vi "Generate Valid Test Numbers.vi"(0 "Session Handle in":T4, 5 "Include All Evaluations?":bool=TRUE, 7 "Test Group":string, 9 "Evaluations In":T1[](array[typedef]) {"Low Limit" format="%#_13g"; "SI Scaling" items=["femto"=-15, "pico"=-12, "nano"=-9, "micro"=-6, "milli"=-3, "percent"=-2, ""=0, "kilo"=3, "mega"=6, "giga"=9, "tera"=12]}, 11 "error in (no error)":errorcluster) -> (4 "Session Handle out":T4, 10 "Evaluations Out":T1[](array[typedef]) {"Low Limit" format="%#_13g"; "SI Scaling" items=["femto"=-15, "pico"=-12, "nano"=-9, "micro"=-6, "milli"=-3, "percent"=-2, ""=0, "kilo"=3, "mega"=6, "giga"=9, "tera"=12]}, 15 "error out":errorcluster)   [LabVIEW 2018, in "Test Number and Bin Generator.lvlib" / "Test Number and Bin Generator.lvclass"]
uses:
  Test Number and Bin Generator.lvclass
  Typedefs/Session Handle.ctl
  Plugins/TestStand API Tools (TSAT).lvlibp/Evaluation Actions/Includes/Controls/TSAT Evaluation.ctl
  Plugins/TestStand API Tools (TSAT).lvlibp/Evaluation Actions/Includes/Controls/TSAT Eval SI Unit Scaling.ctl
  Plugins/TestStand API Tools (TSAT).lvlibp/Evaluation Actions/Includes/Controls/TSAT Evaluation Type.ctl
  Test Number and Bin Generator.lvclass/Test Number and Bin Generator.ctl
  Test Group/Test Group.lvclass
  Test Group/Test Group.lvclass/Test Group.ctl
  Plugins/TestStand API Tools (TSAT).lvlibp/Evaluation Actions/TSAT Evaluation Actions.lvlib
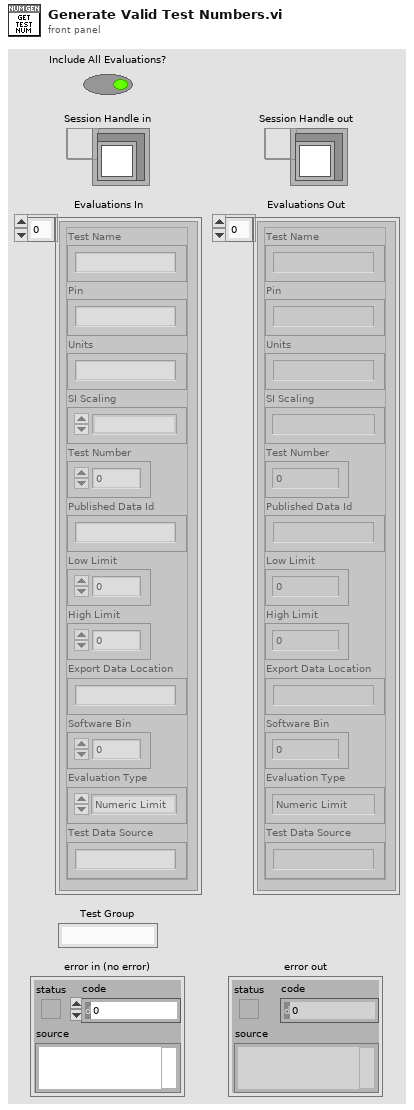
[diagram p1: front panel]
types:
  T1 = typedef "TestStand API Tools (TSAT).lvlibp/TSAT Evaluation Actions.lvlib/TSAT Evaluation.ctl" = cluster{"Test Name":string, "Pin":string, "Units":string, "SI Scaling":T2, "Test Number":i32, "Published Data Id":string, "Low Limit":dbl, "High Limit":dbl, "Export Data Location":string, "Software Bin":i64, "Evaluation Type":T3, "Test Data Source":string}
  T2 = typedef "TestStand API Tools (TSAT).lvlibp/TSAT Evaluation Actions.lvlib/TSAT Eval SI Unit Scaling.ctl" = i16
  T3 = typedef "TestStand API Tools (TSAT).lvlibp/TSAT Evaluation Actions.lvlib/TSAT Evaluation Type.ctl" = enum16{"Numeric Limit", "Pass/Fail", "None"}
  T4 = typedef "Test Number and Bin Generator.lvlib/Test Number and Bin Generator.lvclass/Session Handle.ctl" = refnum<data-value>
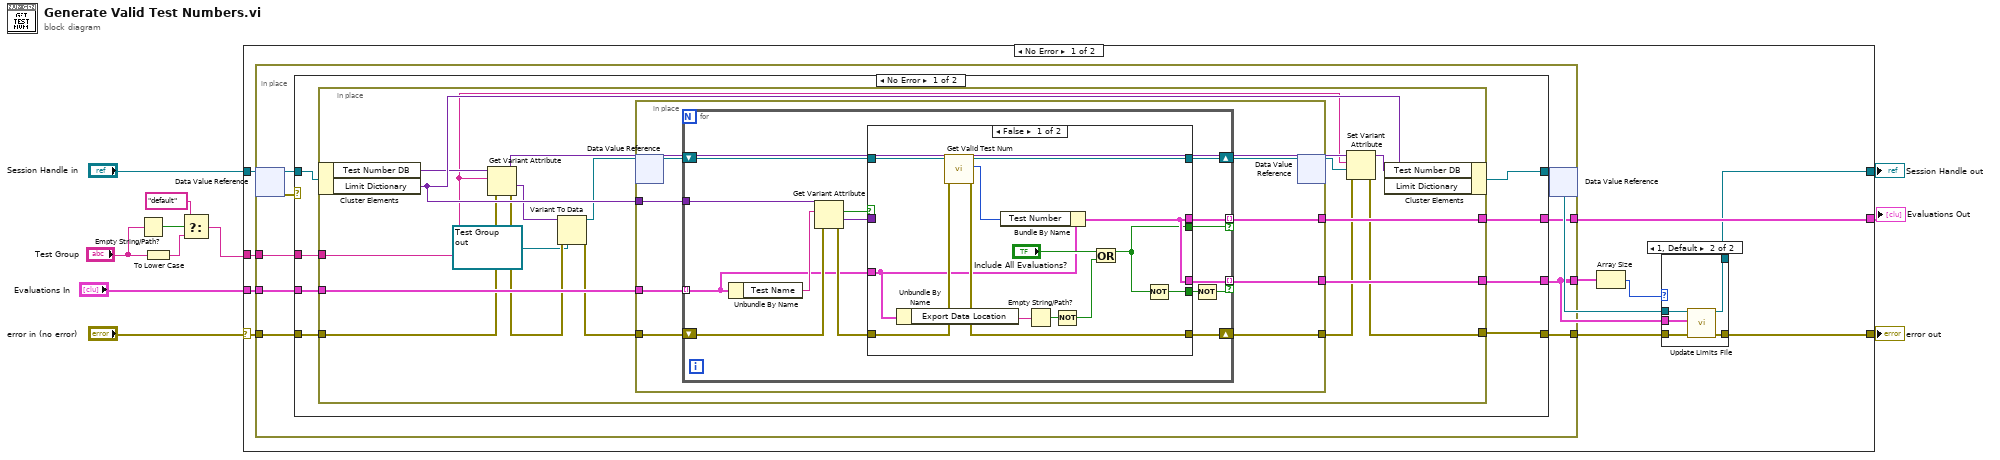
[diagram p0: block diagram]
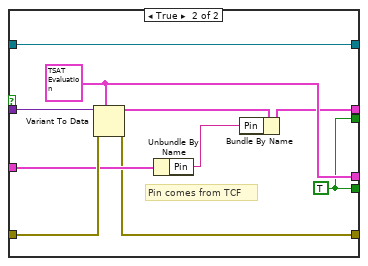
[diagram p3: hidden frame]
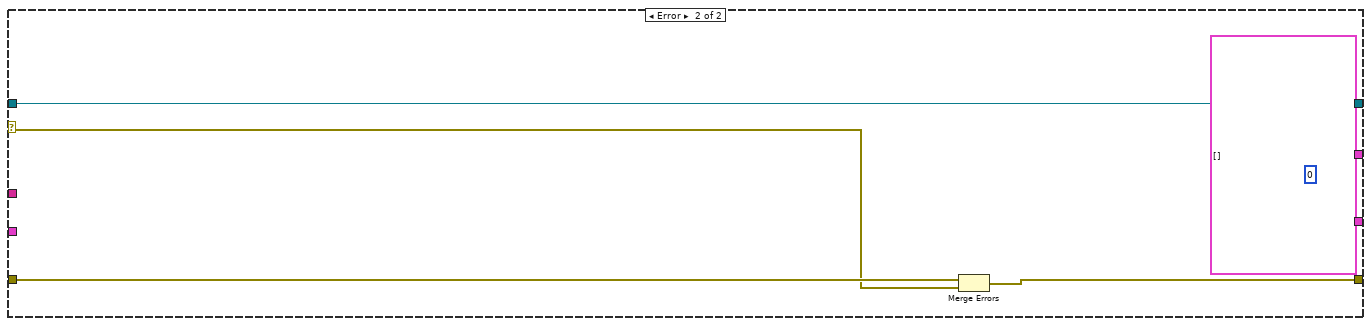
[diagram p4: hidden frame]
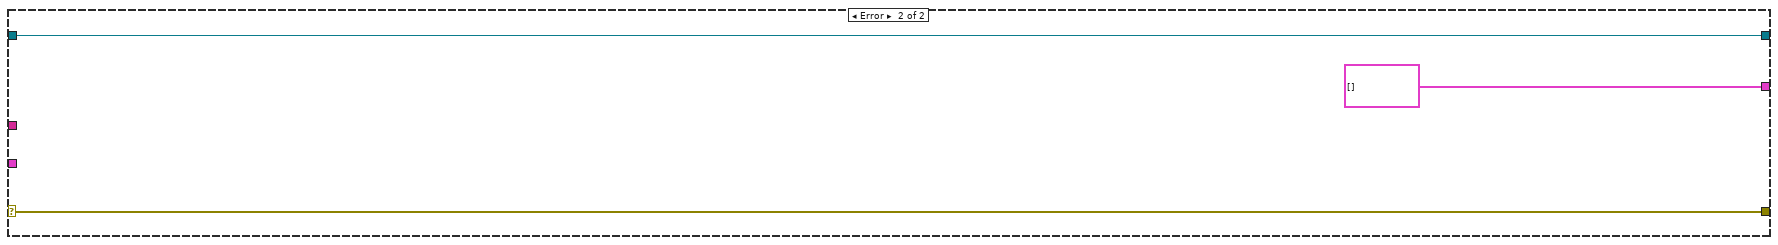
[diagram p5: hidden frame]
diagram:
  n1 = Empty String/Path?(string/path="Test Group") -> (empty?=w5:bool)
  n2 = To Lower Case(string="Test Group") -> (all lower case string=w2:string)
  n3 = Select(t="default", s=w5, f=w2) -> (s? t:f=w1:string)
  n4 = case shown="No Error" "error in (no error)" {
    selector: "error in (no error)" -> [w21 w116]
    tunnel: "Session Handle in" -> [w22 w117]
    tunnel: [w12 w117] -> w10
    tunnel: [w15 w116] -> w9
    tunnel: w1 -> [w20 _]
    tunnel: "Evaluations In" -> [w19 _]
    tunnel: [w18 T1[] []] -> w6
    frame No Error {
      n5 = in-place {
        in-place-border: w21 -> [w34]
        in-place-border: [w37] -> w16
        in-place-border: w20 -> [w33]
        in-place-border: w19 -> [w32]
        in-place-border: [w31] -> w18
        in-place-border: [w30] -> w14
        n6 = in-place-dvr #1(w22) -> (w38:refnum<class "Test Number and Bin Generator.lvclass">, w35:errorcluster)
        n7 = case shown="No Error" w35 {
          selector: w35 -> [_ w113]
          tunnel: w38 -> [w46 w111]
          tunnel: [w42 w112] -> w37
          tunnel: [w45 w111] -> w36
          tunnel: w34 -> [w44 w114]
          tunnel: w33 -> [w43 _]
          tunnel: w32 -> [w41 _]
          tunnel: [w40 w110] -> w31
          tunnel: [w39 w110] -> w30
          frame No Error {
            n8 = in-place {
              in-place-border: w44 -> [w59]
              in-place-border: w43 -> [w49]
              in-place-border: [w53] -> w42
              in-place-border: w41 -> [w63]
              in-place-border: [w62] -> w40
              in-place-border: [w61] -> w39
              n9 = in-place-cluster #2(w46) -> ("Test Number DB"=w58:variant, "Limit Dictionary"=w60:variant)
              n10 = Get Variant Attribute(Variant=w58, name=w49, error in=w59) -> (duplicate Variant=w50:variant, value=w47:variant, error out=w57:errorcluster)  [unwired: 1 in, 1 out]
              n11 = Variant To Data(error in=w57, type=refnum<data-value> refnum ("data value reference"), Variant=w47) -> (data=w55:refnum<data-value>, error out=w56:errorcluster)
              n12 = in-place {
                in-place-border: w63 -> [w71]
                in-place-border: [w70] -> w52
                in-place-border: [w69] -> w62
                in-place-border: [w68] -> w61
                in-place-border: w60 -> [w67]
                in-place-border: w56 -> [w66]
                n13 = in-place-dvr #3(w55) -> (w65:refnum<class "Test Group.lvclass">)  [unwired: 1 out]
                n14 = for {
                  tunnel: w71 -> [w79] mode=indexing
                  shift-right: [w78] -> w70
                  shift-left: w66 -> [w84]
                  tunnel: [w80] -> w69 mode=indexing if=w72
                  tunnel: [w77] -> w68 mode=indexing if=w75
                  tunnel: w67 -> [w86]
                  shift-right: [w73] -> w64
                  shift-left: w65 -> [w74]
                  n15 = Unbundle By Name(w79) -> ("Test Name"=w85:string)
                  n16 = Get Variant Attribute(Variant=w86, name=w85, error in=w84) -> (found=w83:bool, value=w81:variant, error out=w82:errorcluster)  [unwired: 1 in, 1 out]
                  n17 = case shown="False" w83 {
                    tunnel: w82 -> [w95 w107]
                    tunnel: w81 -> [_ w109]
                    tunnel: [w99 w102] -> w80
                    tunnel: w79 -> [w91 w104]
                    tunnel: [w94 w100] -> w78
                    tunnel: [w99 w108] -> w77
                    tunnel: [w92 w105] -> w76
                    tunnel: w74 -> [w98 w106]
                    tunnel: [w96 w106] -> w73
                    tunnel: [w89 w105] -> w72
                    frame False {
                      n18 = Unbundle By Name(w91) -> ("Export Data Location"=w90:string)
                      n19 = call "Get Valid Test Num.vi"("error in (no error)"=w95, "Test Group in"=w98) -> ("error out"=w94:errorcluster, "Numeric"=w97:i32, "Test Group out"=w96:refnum<class "Test Group.lvclass">)  [unwired: 7 in]
                      n20 = Bundle By Name(cluster=w91, "Test Number"=w97) -> (w99:T1)
                      n21 = Empty String/Path?(string/path=w90) -> (empty?=w88:bool)
                      n22 = Not(x=w88) -> (.not. x?=w87:bool)
                      n23 = Or(x="Include All Evaluations?", y=w87) -> (x .or. y?=w89:bool)
                      n24 = Not(x=w89) -> (.not. x?=w92:bool)
                    }
                    frame True {
                      w105 = TRUE
                      w108 = T1 {"Test Name"="", "Pin"="", "Units"="", "SI Scaling"=0, "Test Number"=0, "Published Data Id"="", "Low Limit"=0.0, "High Limit"=0.0, "Export Data Location"="", "Software Bin"=0, "Evaluation Type"=enum."Numeric Limit", "Test Data Source"=""} ("Evaluation")
                      # "Pin comes from TCF"
                      n25 = Variant To Data(error in=w107, type=w108, Variant=w109) -> (data=w103:T1, error out=w100:errorcluster)
                      n26 = Unbundle By Name(w104) -> ("Pin"=w101:string)
                      n27 = Bundle By Name(cluster=w103, "Pin"=w101) -> (w102:T1)
                    }
                  }
                  n28 = Not(x=w76) -> (.not. x?=w75:bool)
                }
                n29 = in-place-dvr #3(w64) -> (w51:refnum<data-value>)  [unwired: 1 out]
              }
              n30 = Set Variant Attribute(Variant=w50, name=w49, value=w51, error in=w52) -> (Variant out=w54:variant, error out=w53:errorcluster)  [unwired: 1 out]
              n31 = in-place-cluster #2("Test Number DB"=w54, "Limit Dictionary"=w60) -> (w45:refnum<class "Test Number and Bin Generator.lvclass">)
            }
          }
          frame Error {
            w110 = T1[] []
            (unwired) 0 ("Entry Value")
            n32 = Merge Errors(w114, w113) -> (w112:errorcluster)
          }
        }
        n33 = in-place-dvr #1(w36) -> (w17:T4)  [unwired: 1 out]
      }
      n34 = Array Size(array=w14) -> (size(s)=w13:i32)
      n35 = case shown="1, Default" w13 {
        tunnel: w17 -> [w23 w29]
        tunnel: w16 -> [w24 w27]
        tunnel: [w24 w26] -> w15
        tunnel: w14 -> [_ w25]
        tunnel: [w23 w28] -> w12
        frame 0 {
        }
        frame 1, Default {
          n36 = call "Update Limits File.vi"("Session Handle in"=w29, "Evaluations In"=w25, "error in (no error)"=w27) -> ("Session Handle out"=w28:T4, "error out"=w26:errorcluster)  [unwired: 11 in]
        }
      }
    }
    frame Error {
    }
  }
  "Session Handle out" <- w10
  "error out" <- w9
  "Evaluations Out" <- w6
